vi "Bool to string.vi"(11 "Autoreturn":bool) -> (3 "Peak app":string)   [LabVIEW 2019, in "STAV lib.lvlib"]
uses:
  STAV lib.lvlib
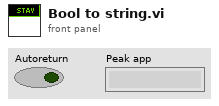
[diagram p1: front panel]
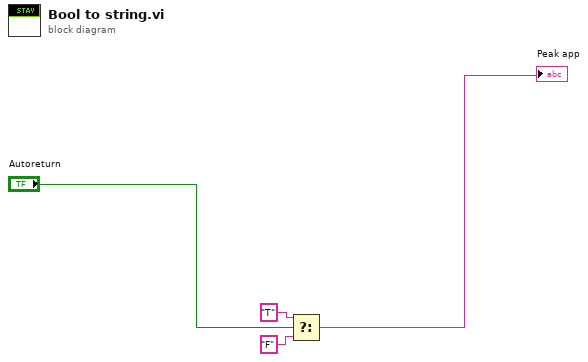
[diagram p0: block diagram]
diagram:
  n1 = Select(t="T" ("Peak app"), s="Autoreturn", f="F" ("Peak app")) -> (s? t:f=→"Peak app":string)
